vi "AES Release.vi"(8 "error in (no error)":errorcluster, 11 "AES in":refnum<class "AES.lvclass">) -> (0 "error out":errorcluster)   [LabVIEW 2023, in "AES.lvclass"]
uses:
  AES.lvclass
  AES.lvclass/AES.ctl
  System.Core
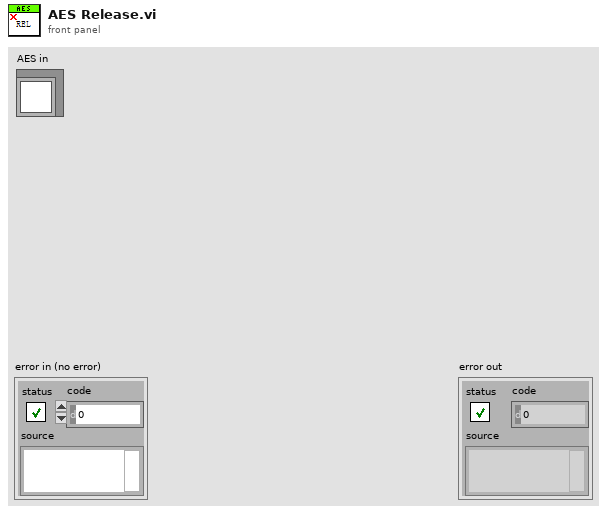
[diagram p1: front panel]
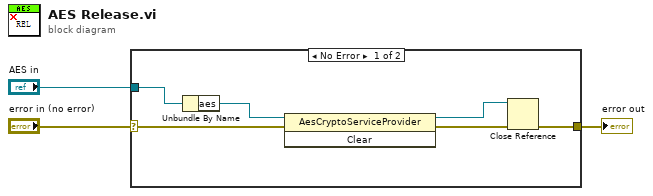
[diagram p0: block diagram]
diagram:
  n1 = case shown="No Error" "error in (no error)" {
    selector: "error in (no error)" -> [w8 w10]
    tunnel: [w4 w10] -> w2
    tunnel: "AES in" -> [w9 _]
    frame No Error {
      n2 = Unbundle By Name(w9) -> ("aes"=w7:refnum<k24>)
      n3 = invoke class="AesCryptoServiceProvider" method="Clear"(reference=w7, error in=w8) -> (reference out=w5:refnum<k24>, error out=w6:errorcluster)  [unwired: 1 in, 1 out]
      n4 = Close Reference(reference=w5, error in (no error)=w6) -> (error out=w4:errorcluster)
    }
    frame Error {
    }
  }
  "error out" <- w2
